vi "Draw Circle.vi"(6 "IoU":sgl=0.45, 8 "threshold":sgl=0.9 format="%#_13g", 9 "dim":i64[](array[numeric])=[1, 5, 21504], 10 "data":sgl[](array[numeric]), 11 "image in":picture) -> (1 "Circles":cluster{"x":sgl, "y":sgl, "r":sgl}[](array[cluster]), 2 "count":i32, 3 "image out":picture)   [LabVIEW 2017, in "postprocess_YOLOv8.lvlib"]
uses:
  postprocess_YOLOv8.lvlib
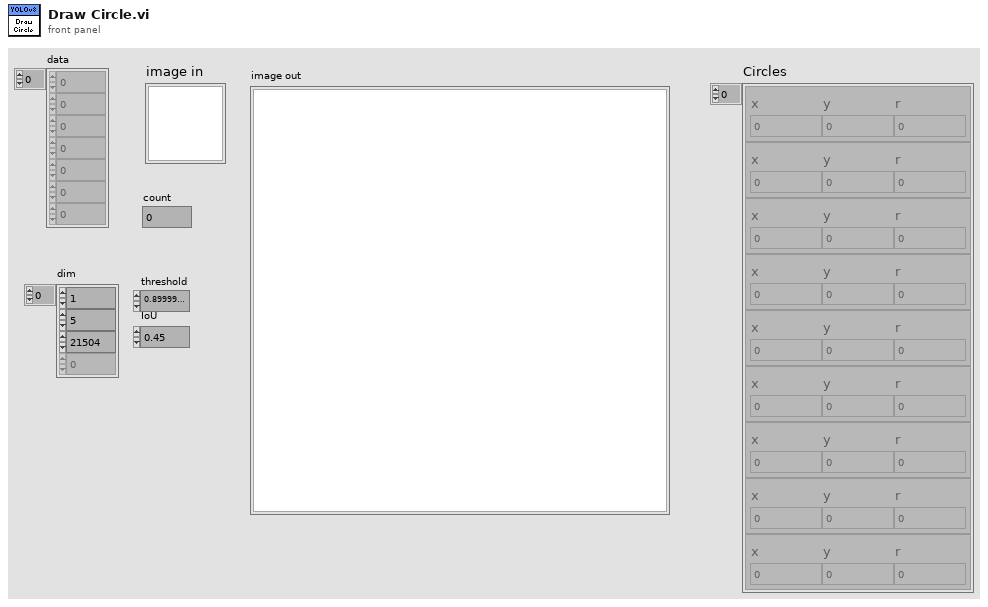
[diagram p1: front panel]
types:
  T1 = typedef "postprocess_YOLOv8.lvlib/Box.ctl" = cluster{"conf":sgl, "x_center":sgl, "y_center":sgl, "width":sgl, "height":sgl, "x1":sgl, "y1":sgl, "x2":sgl, "y2":sgl}
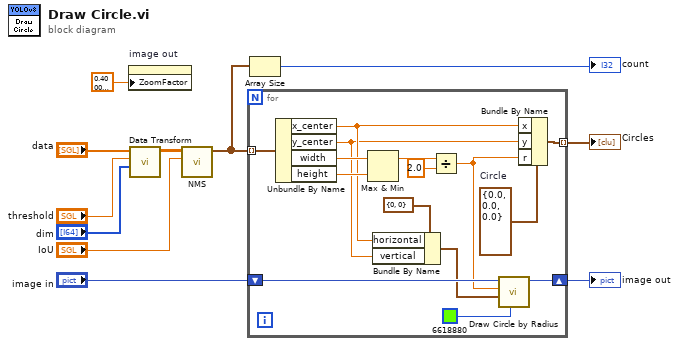
[diagram p0: block diagram]
diagram:
  n1 = property on="image out" class="Pict"("ZoomFactor"=sgl 0.4 ("Zoom Factor")) -> ()  [unwired: 2 in, 2 out]
  n2 = call "Data Transform.vi"("dim"="dim", "threshold"="threshold", "Array in"="data") -> ("Array out"=w8:sgl[][])  [unwired: 8 in]
  n3 = call "NMS.vi"("IoU"="IoU", "Array in"=w8) -> ("Box out"=w6:T1[])  [unwired: 9 in]
  n4 = for {
    shift-right: [w25] -> w10
    shift-left: "image in" -> [w26]
    tunnel: w6 -> [w21] mode=indexing
    tunnel: [w12] -> w2 mode=indexing
    w16 = cluster{"x":sgl, "y":sgl, "r":sgl} {"x"=0.0, "y"=0.0, "r"=0.0}  # Circle
    n5 = Unbundle By Name(w21) -> ("x_center"=w15:sgl, "y_center"=w14:sgl, "width"=w20:sgl, "height"=w19:sgl)
    n6 = Max & Min(x=w20, y=w19) -> (max(x,y)=w18:sgl)  [unwired: 1 out]
    n7 = Bundle By Name(cluster=cluster{"horizontal":i16, "vertical":i16} {"horizontal"=0, "vertical"=0} ("pixel center"), "horizontal"=w15, "vertical"=w14) -> (w22:cluster{"horizontal":i16, "vertical":i16})
    n8 = Divide(x=w18, y=sgl 2.0) -> (x/y=w13:sgl)
    n9 = call <vilib>:"Draw Circle by Radius.vi"("color(black)"=u32 6618880, "pixel center"=w22, "radius"=w13, "picture"=w26) -> ("new picture"=w25:picture)  [unwired: 7 in]
    n10 = Bundle By Name(cluster=w16, "x"=w15, "y"=w14, "r"=w13) -> (w12:cluster{"x":sgl, "y":sgl, "r":sgl})
  }
  "image out" <- w10
  "Circles" <- w2
  n11 = Array Size(array=w6) -> (size(s)=→"count":i32)
